vi "Find This Level Leaves.vi"(8 "error in":errorcluster, 11 "Tree in":refnum<class "Tree.lvclass">) -> (0 "error out":errorcluster, 1 "Values":variant[](array[variant]), 2 "Keys":string[](array[string]), 3 "Tree out":refnum<class "Tree.lvclass">)   [LabVIEW 2019, in "Tree.lvclass"]
uses:
  Tree.lvclass
  Tree.lvclass/Tree.ctl
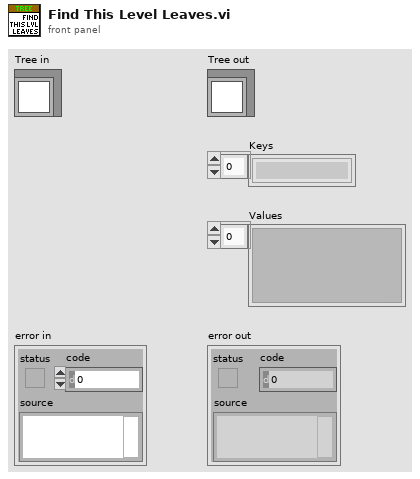
[diagram p1: front panel]
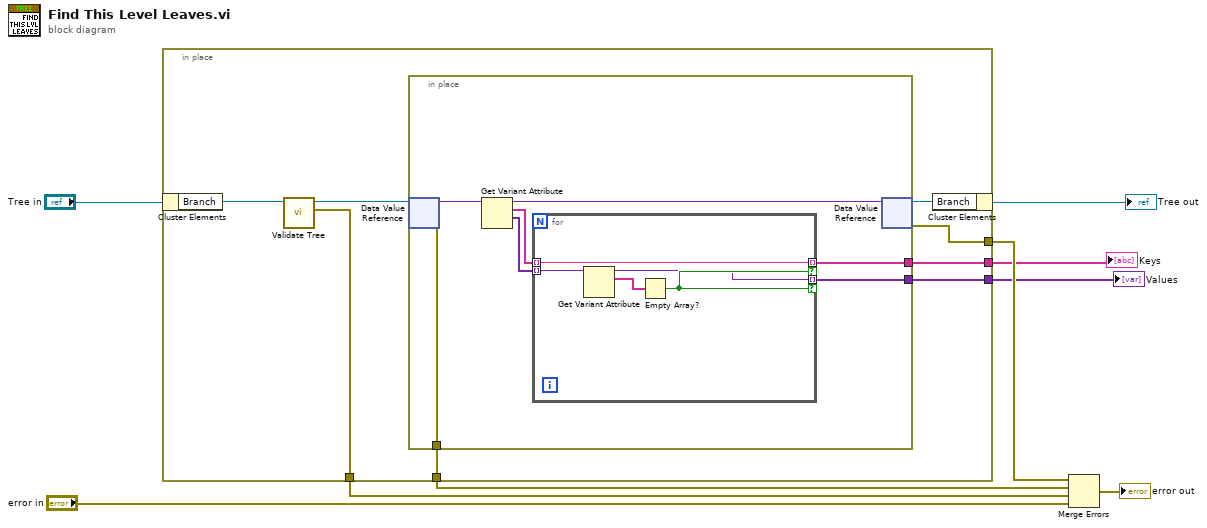
[diagram p0: block diagram]
diagram:
  n1 = in-place {
    in-place-border: [w16] -> w5
    in-place-border: [w10] -> w3
    in-place-border: [w15] -> w4
    in-place-border: [w14] -> w2
    in-place-border: [w13] -> w1
    n2 = in-place-cluster #1("Tree in") -> ("Branch"=w12:refnum<data-value>)
    n3 = call "Validate Tree.vi"("Branch Reference In"=w12) -> ("error out"=w10:errorcluster, "Branch Reference Out"=w11:refnum<data-value>)  [unwired: 9 in]
    n4 = in-place {
      in-place-border: [w24] -> w15
      in-place-border: [w19] -> w14
      in-place-border: [w18] -> w13
      n5 = in-place-dvr #2(w11) -> (w23:variant, w24:errorcluster)
      n6 = Get Variant Attribute(Variant=w23) -> (duplicate Variant=w22:variant, names=w21:string[], values=w20:variant[])  [unwired: 3 in, 1 out]
      n7 = for {
        tunnel: w21 -> [w27] mode=indexing
        tunnel: w20 -> [w29] mode=indexing
        tunnel: [w27] -> w19 mode=indexing if=w26
        tunnel: [w25] -> w18 mode=indexing if=w26
        n8 = Get Variant Attribute(Variant=w29) -> (duplicate Variant=w25:variant, names=w28:string[])  [unwired: 3 in, 2 out]
        n9 = Empty Array?(array=w28) -> (empty?=w26:bool)
      }
      n10 = in-place-dvr #2(w22) -> (w17:refnum<data-value>, w16:errorcluster)
    }
    n11 = in-place-cluster #1("Branch"=w17) -> (→"Tree out":refnum<class "Tree.lvclass">)
  }
  "Values" <- w1
  "Keys" <- w2
  n12 = Merge Errors(w5, w4, w3, "error in") -> (→"error out":errorcluster)
